vi "RFController SetTriggerWait.vi"(6 "contextId":T1, 8 "error in":errorcluster, 9 "timeout (ms)":i32=-1, 10 "Request Data":T3, 11 "gRPC ID":T1) -> (0 "error out":errorcluster, 2 "Response Data":T2, 3 "gRPC ID out":T1)   [LabVIEW 2024, in "FlexSDR_gRPC_client.lvlib"]
uses:
  FlexSDR_gRPC_client.lvlib
  <vilib>/gRPC/LabVIEW gRPC Library/Shared/grpcId.ctl
  RPC Messages/rfcontrol_SetTriggerWaitRequest.ctl
  RPC Messages/rfcontrol_SetTriggerWaitResponse.ctl
  RPC Messages/rfcontrol_SetTriggerWaitResponse_Flat.ctl
  14035477-4c25-4107-8ed5-d0c4ef420ce5.vi
  <vilib>/gRPC/LabVIEW gRPC Library/Shared/TranslateGrpcError.vi
  <vilib>/gRPC/LabVIEW gRPC Library/Shared/Wait On Occurrence.vi
  <vilib>/gRPC/LabVIEW gRPC Library/Shared/Is Feature Enabled.vi
  <vilib>/gRPC/LabVIEW gRPC Library/Server API/Server/Get Server DLL Path.vi
  <vilib>/Utility/error.llb/Error Cluster From Error Code.vi
  <vilib>/gRPC/LabVIEW gRPC Library/grpc-lvsupport-release.lvlib
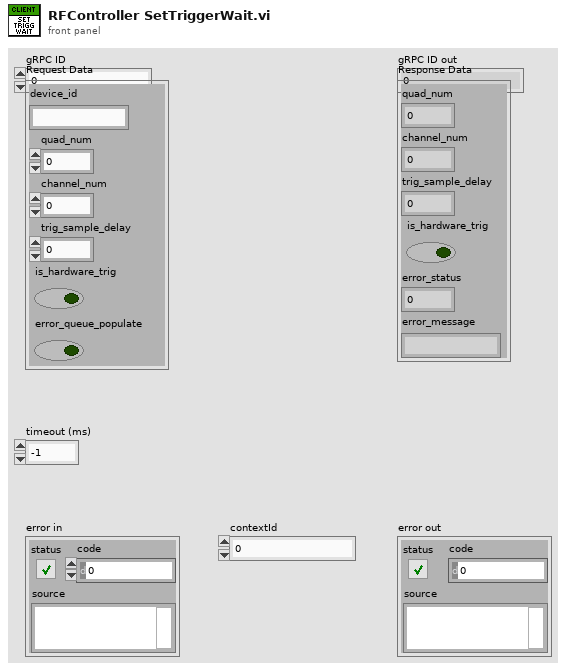
[diagram p1: front panel]
types:
  T1 = typedef "grpc-lvsupport-release.lvlib/grpcId.ctl" = u64
  T2 = typedef "FlexSDR_gRPC_client.lvlib/rfcontrol_SetTriggerWaitResponse.ctl" = cluster{"quad_num":i32, "channel_num":i32, "trig_sample_delay":i32, "is_hardware_trig":bool, "error_status":i32, "error_message":string}
  T3 = typedef "FlexSDR_gRPC_client.lvlib/rfcontrol_SetTriggerWaitRequest.ctl" = cluster{"device_id":string, "quad_num":i32, "channel_num":i32, "trig_sample_delay":i32, "is_hardware_trig":bool, "error_queue_populate":bool}
  T4 = typedef "FlexSDR_gRPC_client.lvlib/rfcontrol_SetTriggerWaitResponse_Flat.ctl" = cluster{"quad_num":i32, "channel_num":i32, "trig_sample_delay":i32, "is_hardware_trig":bool, "error_status":i32, "error_message":string}
  T5 = typedef "FlexSDR_gRPC_client.lvlib/rfcontrol_SetTriggerWaitRequest_Flat.ctl" = cluster{"device_id":string, "quad_num":i32, "channel_num":i32, "trig_sample_delay":i32, "is_hardware_trig":bool, "error_queue_populate":bool}
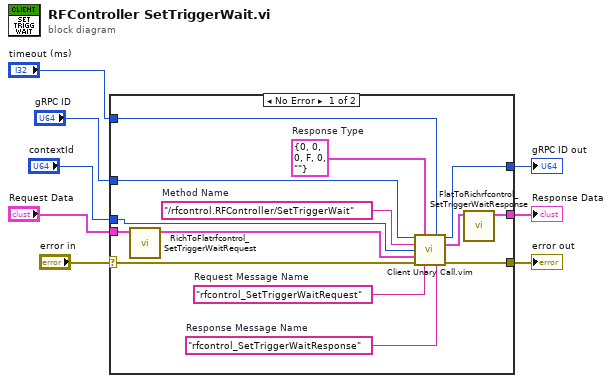
[diagram p0: block diagram]
diagram:
  n1 = case shown="No Error" "error in" {
    selector: "error in" -> [w18 w23]
    tunnel: [w17 w23] -> w7
    tunnel: "gRPC ID" -> [w16 w24]
    tunnel: [w15 w24] -> w5
    tunnel: "Request Data" -> [w12 _]
    tunnel: [w9 _] -> w3
    tunnel: "timeout (ms)" -> [w14 _]
    tunnel: "contextId" -> [w13 _]
    frame No Error {
      w19 = "rfcontrol_SetTriggerWaitResponse"  # Response Message Name
      w20 = "rfcontrol_SetTriggerWaitRequest"  # Request Message Name
      w21 = T4 {"quad_num"=0, "channel_num"=0, "trig_sample_delay"=0, "is_hardware_trig"=FALSE, "error_status"=0, "error_message"=""}  # Response Type
      w22 = "/rfcontrol.RFController/SetTriggerWait"  # Method Name
      n2 = call "RichToFlatrfcontrol_SetTriggerWaitRequest.vi"("InputCluster"=w12) -> ("OutputCluster"=w11:T5)  [unwired: 10 in]
      n3 = call "Client Unary Call.vim"("ClientID in"=w16, "Response Type"=w21, "timeout (ms)"=w14, "Method Name"=w22, "contextId"=w13, "Request Data"=w11, "error in"=w18, "Request Message Name"=w20, "Response Message Name"=w19) -> ("ClientID out"=w15:u64, "Response Data"=w10:T4, "error out"=w17:errorcluster)  [unwired: 4 in]
      n4 = call "FlatToRichrfcontrol_SetTriggerWaitResponse.vi"("InputCluster"=w10) -> ("OutputCluster"=w9:T2)  [unwired: 10 in]
    }
    frame Error {
    }
  }
  "error out" <- w7
  "gRPC ID out" <- w5
  "Response Data" <- w3
